vi "str to timestamp.vi"(1 "date/time string":string) -> (0 "Resulting Time Stamp":timestamp)   [LabVIEW 2013, in "CreateOPCUAServerAuto.lvlib"]
doc: "This VI convert a date/time string back to a time stamp."
uses:
  CreateOPCUAServerAuto.lvlib
panel:
  # "This control should have data in the form:\n4/30/2004 7:48:47 PM"
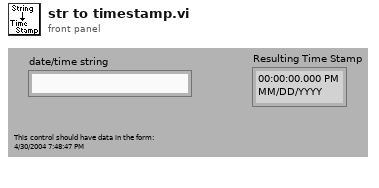
[diagram p1: front panel]
types:
  T1 = cluster{"second":i32, "minute":i32, "hour":i32, "day of month":i32, "month":i32, "year":i32, "day of week":i32, "day of year":i32, "is DST":i32}
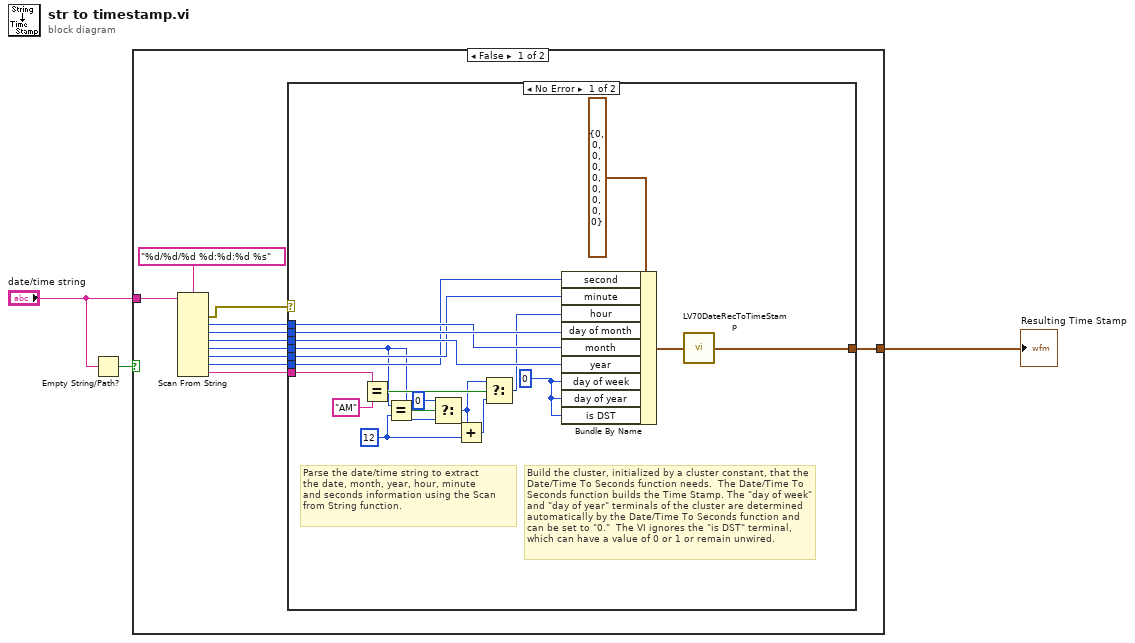
[diagram p0: block diagram]
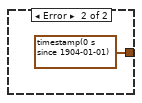
[diagram p2: hidden frame]
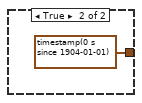
[diagram p3: hidden frame]
diagram:
  n1 = Empty String/Path?(string/path="date/time string") -> (empty?=w1:bool)
  n2 = case shown="False" w1 {
    tunnel: "date/time string" -> [w6 _]
    tunnel: [w5 timestamp(0 s since 1904-01-01) ("Time Stamp")] -> w2
    frame False {
      n3 = Scan From String "Scan From String"(format string="%d/%d/%d %d:%d:%d %s", input string=w6) -> (error out=w4:errorcluster, output 1=w12:i32, output 2=w13:i32, output 3=w11:i32, output 4=w7:i32, output 5=w10:i32, output 6=w9:i32, output 7=w8:string)  [unwired: 9 in, 2 out]
      n4 = case shown="No Error" w4 {
        tunnel: w13 -> [w30 _]
        tunnel: w12 -> [w29 _]
        tunnel: w11 -> [w28 _]
        tunnel: w10 -> [w27 _]
        tunnel: w9 -> [w26 _]
        tunnel: w8 -> [w25 _]
        tunnel: w7 -> [w18 _]
        tunnel: [w15 timestamp(0 s since 1904-01-01) ("Time Stamp")] -> w5
        frame No Error {
          w20 = 12 ("y")
          w31 = 0
          # "Build the cluster, initialized by a cluster constant, that the Date/Time To Seconds function needs.  The Date/Time To Seconds function builds the Time Stamp. The \"day of week\" and \"day of year\" terminals of the cluster are determined automatically by the Date/Time To Seconds function and can be set to \"0.\"  The VI ignores the \"is DST\" terminal, which can have a value of 0 or 1 or remain unwired."
          # "Parse the date/time string to extract \nthe date, month, year, hour, minute \nand seconds information using the Scan\nfrom String function."
          n5 = Equal?(x=w25, y="AM") -> (x = y?=w21:bool)
          n6 = Equal?(x=w18, y=w20) -> (x = y?=w19:bool)
          n7 = Select(t=0, s=w19, f=w18) -> (s? t:f=w17:i32)
          n8 = Add(x=w17, y=w20) -> (x+y=w22:i32)
          n9 = Select(t=w17, s=w21, f=w22) -> (s? t:f=w23:i32)
          n10 = Bundle By Name(cluster=T1 {"second"=0, "minute"=0, "hour"=0, "day of month"=0, "month"=0, "year"=0, "day of week"=0, "day of year"=0, "is DST"=0} ("date time rec"), "second"=w26, "minute"=w27, "hour"=w23, "day of month"=w30, "month"=w29, "year"=w28, "day of week"=w31, "day of year"=w31, "is DST"=w31) -> (w32:T1)
          n11 = call <vilib>:"LV70DateRecToTimeStamp.vi"("date time rec"=w32) -> ("Time Stamp"=w15:timestamp)
        }
        frame Error {
        }
      }
    }
    frame True {
    }
  }
  "Resulting Time Stamp" <- w2
